vi "ESP8266_Wifi_LED_LabVIEW.vi"() -> ()   [LabVIEW 2018]
uses:
  <vilib>/httpClient/POSTBuffer.vi
  <vilib>/httpClient/LabVIEWHTTPClient.lvlib
panel:
  out "ON Button TimeStamp":timestamp
  out "OFF Button TimeStamp":timestamp
  out "Ciklus":i32
  out "Led":bool
  out "field1 read":dbl
  out "value":T1
  in  "Format ref cluster":T1
  in  "OFF Button":bool
  in  "ON Button":bool
  out "body":string
  in  "stop":bool
  in  "milliseconds to wait":u32=1000
  out "headers":string
  # "192.168.0.161"
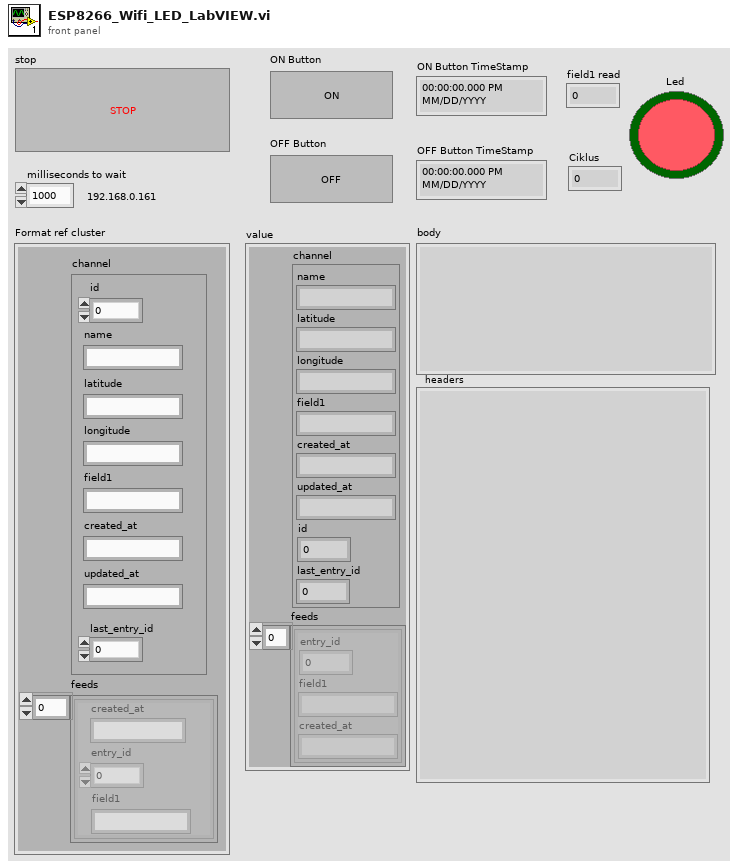
[diagram p1: front panel]
types:
  T1 = cluster{"channel":cluster{"name":string, "latitude":string, "longitude":string, "field1":string, "created_at":string, "updated_at":string, "id":dbl, "last_entry_id":dbl}, "feeds":cluster{"entry_id":dbl, "field1":string, "created_at":string}[]}
  T2 = typedef "LabVIEWHTTPClient.lvlib/ClientHandle.ctl" = refnum<k1>
  T3 = cluster{"entry_id":dbl, "field1":string, "created_at":string}[]
  T4 = cluster{"entry_id":dbl, "field1":string, "created_at":string}
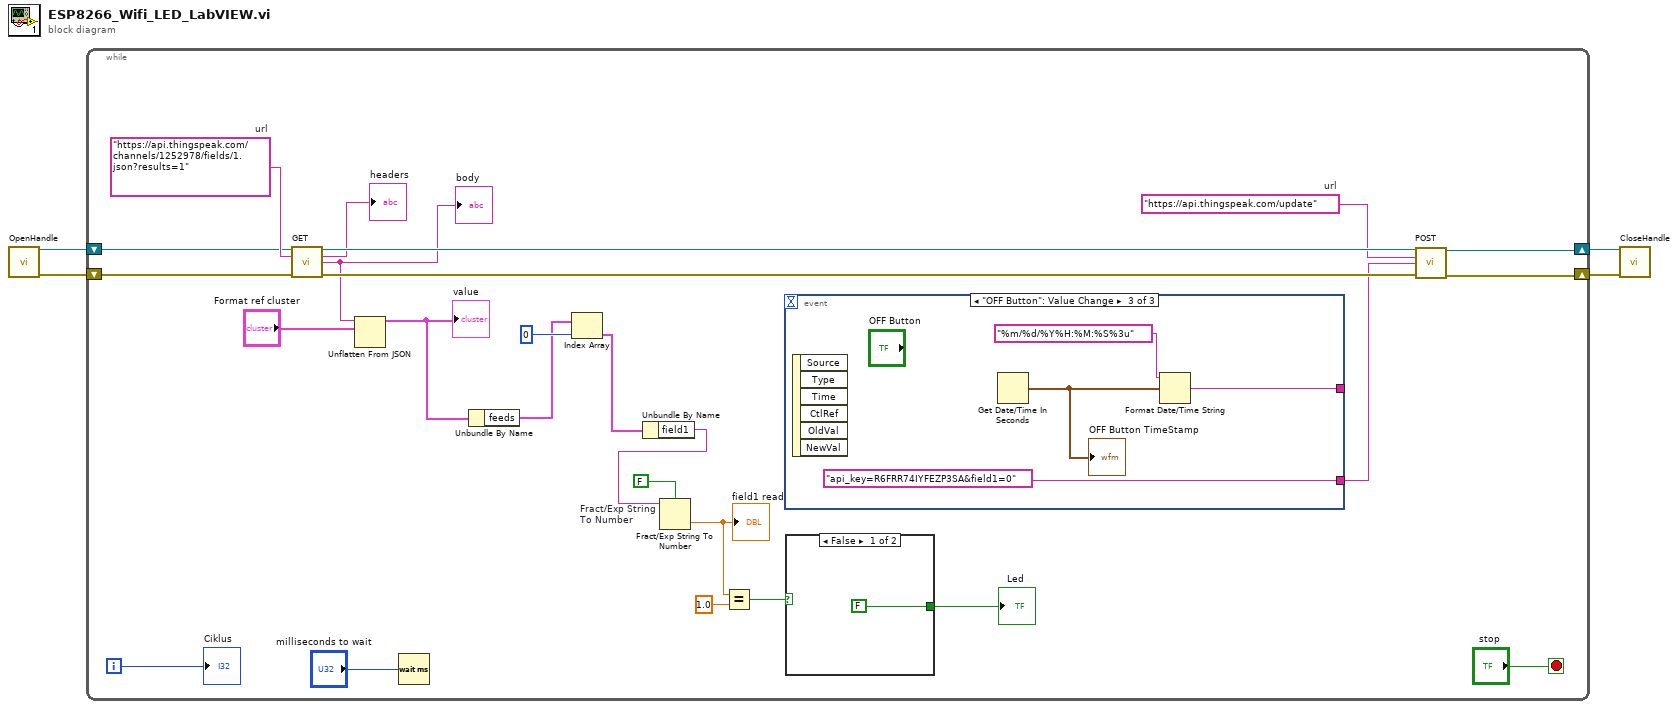
[diagram p0: block diagram]
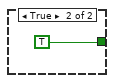
[diagram p2: hidden frame]
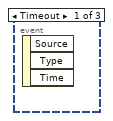
[diagram p3: hidden frame]
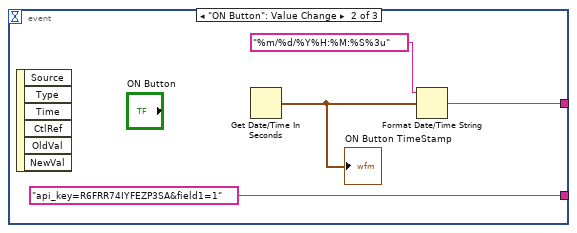
[diagram p4: hidden frame]
diagram:
  n1 = call <vilib>:"OpenHandle.vi"() -> ("client handle out"=w4:T2, "error out"=w3:errorcluster)  [unwired: 14 in]
  n2 = while {
    shift-right: [w19] -> w2
    shift-left: w4 -> [w25]
    shift-right: [w18] -> w1
    shift-left: w3 -> [w24]
    i -> [w6]
    stop <- "stop" stop-if-true
    w26 = "https://api.thingspeak.com/channels/1252978/fields/1.json?results=1"  # url
    w21 = "https://api.thingspeak.com/update"  # url
    n3 = call <vilib>:"GET.vi"("client handle"=w25, "url"=w26, "error in (no error)"=w24) -> ("client handle out"=w23:T2, "headers"=→"headers":string, "body"=w7:string, "error out"=w22:errorcluster)  [unwired: 9 in]
    "body" <- w7
    n4 = Unflatten From JSON(JSON string=w7, type and defaults="Format ref cluster") -> (value=w14:T1)  [unwired: 5 in, 1 out]
    "value" <- w14
    n5 = Wait (ms)(milliseconds to wait="milliseconds to wait") -> ()  [unwired: 1 out]
    n6 = Unbundle By Name "Unbundle By Name"(w14) -> ("feeds"=w15:T3)
    n7 = Index Array "Index Array"(array=w15, index=0) -> (element=w13:T4)
    n8 = Unbundle By Name "Unbundle By Name"(w13) -> ("field1"=w11:string)
    n9 = Fract/Exp String To Number "Fract/Exp String \nTo Number"(use system decimal point (T)=FALSE, string=w11) -> (number=w9:dbl)  [unwired: 2 in, 1 out]
    "field1 read" <- w9
    n10 = Equal?(x=w9, y=1.0) -> (x = y?=w10:bool)
    n11 = event shown="[2] \"OFF Button\": Value Change" {
      selector: _ -> [_ _ _]
      dyn-events: _ -> [_ _ _]
      timeout: _ -> [_ _ _]
      tunnel: [_ "api_key=R6FRR74IYFEZP3SA&field1=1" ("buffer") "api_key=R6FRR74IYFEZP3SA&field1=0" ("buffer")] -> w20
      tunnel: [_ w32 w36] -> _
      event Timeout {
        n12 = event-data() -> ()  [unwired: 1 in, 3 out]
      }
      event "ON Button": Value Change {
        n13 = event-data() -> ()  [unwired: 1 in, 6 out]
        n14 = Get Date/Time In Seconds() -> (seconds since 1Jan1904=w33:timestamp)
        "ON Button TimeStamp" <- w33
        n15 = Format Date/Time String(time format string (%c)="%m/%d/%Y%H:%M:%S%3u", seconds (now)=w33) -> (date/time string=w32:string)  [unwired: 1 in]
      }
      event "OFF Button": Value Change {
        n16 = event-data() -> ()  [unwired: 1 in, 6 out]
        n17 = Get Date/Time In Seconds() -> (seconds since 1Jan1904=w37:timestamp)
        "OFF Button TimeStamp" <- w37
        n18 = Format Date/Time String(time format string (%c)="%m/%d/%Y%H:%M:%S%3u", seconds (now)=w37) -> (date/time string=w36:string)  [unwired: 1 in]
      }
    }
    n19 = case shown="False" w10 {
      tunnel: [FALSE ("Boolean") TRUE ("Boolean")] -> w5
      frame False {
      }
      frame True {
      }
    }
    "Led" <- w5
    n20 = call-poly <vilib>:"POST.vi"("client handle"=w23, "url"=w21, "buffer"=w20, "error in (no error)"=w22) -> ("client handle out"=w19:T2, "error out"=w18:errorcluster)  [unwired: 8 in, 2 out]
    "Ciklus" <- w6
  }
  n21 = call <vilib>:"CloseHandle.vi"("client handle"=w2, "error in (no error)"=w1) -> ()  [unwired: 13 in, 1 out]
